vi "Удаление паузы.vi"() -> ()   [LabVIEW 2017]
panel:
  out "Array":dbl[](array[numeric])
  out "Массив с паузами":dbl[](array[numeric])
  in  "Сколько битов брать":i32=4
  in  "Количество бит":i32=8
  out "Вырезка из массива":dbl[](array[numeric])
  out "Биты на выходе 1":dbl[](array[numeric])
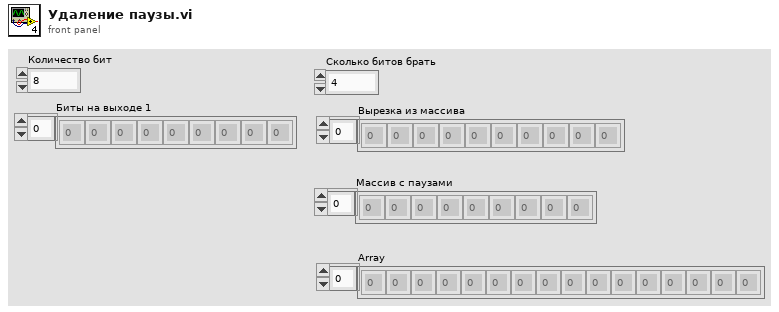
[diagram p1: front panel]
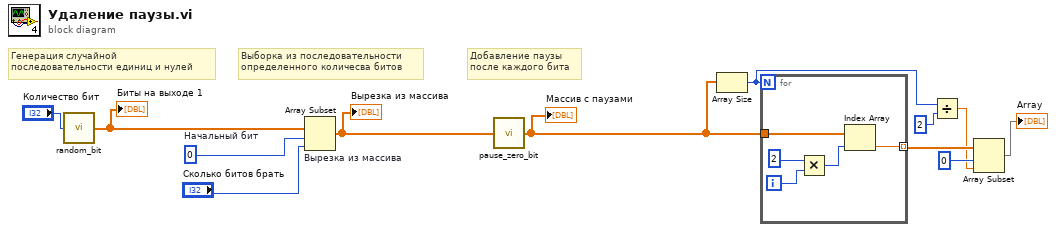
[diagram p0: block diagram]
diagram:
  w12 = 0  # Начальный бит
  # "Добавление паузы \nпосле каждого бита"
  # "Выборка из последовательности\nопределенного количесва битов"
  # "Генерация случайной \nпоследовательности единиц и нулей"
  n1 = call "random_bit.vi"("Количество бит"="Количество бит") -> ("Биты на выходе 1"=w10:dbl[])
  "Биты на выходе 1" <- w10
  n2 = Array Subset "Вырезка из массива"(array=w10, index=w12, length="Сколько битов брать") -> (w8:dbl[])
  "Вырезка из массива" <- w8
  n3 = call "pause_zero_bit.vi"("Входная последовательность"=w8) -> ("Массив с паузами"=w7:dbl[])
  "Массив с паузами" <- w7
  n4 = Array Size(array=w7) -> (size(s)=w4:i32)
  n5 = for {
    N: w4 -> [_]
    tunnel: w7 -> [w17]
    tunnel: [w14] -> w6 mode=indexing
    i -> [w15]
    n6 = Multiply(x=2, y=w15) -> (x*y=w13:i32)
    n7 = Index Array(array=w17, index=w13) -> (element=w14:dbl)
  }
  n8 = Divide(x=w4, y=2) -> (x/y=w2:dbl)
  n9 = Array Subset(array=w6, index=0, length=w2) -> (→"Array":dbl[])
